vi "Teleop.vi"(10 "Match Info":T1={"Autonomous Elapsed Seconds"=0.0, "TeleOp Elapsed Seconds"=0.0, "Disabled Elapsed Seconds"=0.0, "Visited Autonomous"=FALSE, "Visited TeleOp"=FALSE, "Visited Disabled"=FALSE, "Autonomous Settings"={"Autonomous Style"=enum."Independent", "VI Refnum"=refnum}}, 11 "Call Context":T2) -> ()   [LabVIEW 2016]
doc: "This VI is called for each TeleOp packet received from the DS where the robot is not disabled. It is often used to read from the joysticks and update I/O or to update setpoints for timed control loops. It should complete and return within 20 milliseconds or it may miss DS packets."
uses:
  <vilib>/Rock Robotics/WPI/DriverStation/WPI_DriverStationDerivedRobotMode.ctl
  <vilib>/Rock Robotics/WPI/DriverStation/WPI_DriverStationMatch Info.ctl
  <vilib>/Rock Robotics/WPI/Utilities/WPI_GetSetVariantRefNum.vi
  <vilib>/Rock Robotics/Network Tables/NT Write Boolean Array.vi
  <vilib>/Rock Robotics/Network Tables/NT Write Numeric Array.vi
  <vilib>/Rock Robotics/Network Tables/NT Read Boolean.vi
  <vilib>/Rock Robotics/Network Tables/NT Read Number.vi
  Robot Global Data.vi
  <vilib>/Rock Robotics/WPI/RobotDrive/WPI_RobotDriveArcadeDrive_Standard(NoSaturation).vi
panel:
  out "Sample Slider 0":dbl(slide) scale=0.0..5.0
  out "Sample Boolean 1":bool
  out "Sample Boolean 0":bool
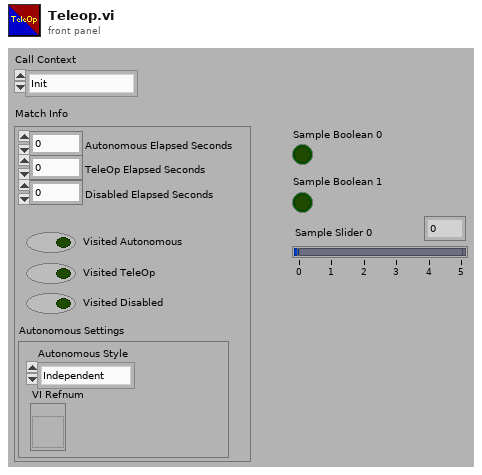
[diagram p1: front panel]
types:
  T1 = typedef "WPI_DriverStationMatch Info.ctl" = cluster{"Autonomous Elapsed Seconds":dbl, "TeleOp Elapsed Seconds":dbl, "Disabled Elapsed Seconds":dbl, "Visited Autonomous":bool, "Visited TeleOp":bool, "Visited Disabled":bool, "Autonomous Settings":cluster{"Autonomous Style":enum16{"Iterative", "Independent"}, "VI Refnum":refnum<vi>}}
  T2 = typedef "WPI_DriverStationDerivedRobotMode.ctl" = enum16{"Init", "Execute", "Stop"}
  T3 = typedef "WPI_JoystickDevRef.ctl" = cluster{"Device":T4}
  T4 = typedef "WPI_JoystickDeviceEnum.ctl" = enum16{"USB 0", "USB 1", "USB 2", "USB 3", "USB 4", "USB 5"}
  T5 = cluster{"Axes[0]":dbl, "Axes[1]":dbl, "Axes[2]":dbl, "Axes[3]":dbl, "Axes[4]":dbl, "Axes[5]":dbl, "Axes[6]":dbl, "Axes[7]":dbl, "Axes[8]":dbl}
  T6 = cluster{"Buttons[0]":bool, "Buttons[1]":bool, "Buttons[2]":bool, "Buttons[3]":bool, "Buttons[4]":bool, "Buttons[5]":bool, "Buttons[6]":bool, "Buttons[7]":bool, "Buttons[8]":bool}
  T7 = typedef "WPI_MotorControlDeviceRef.ctl" = cluster{"DeviceStatus":errorcluster, "Type":T8, "PWM":cluster{"PWM Channel":T9, "DeadBand":T10}, "CAN":cluster{"Device Number":u8, "SetOutput VI Ref":variant, "GetOutput VI Ref":variant, "Enable VI Ref":variant, "Disable VI Ref":variant, "Data":variant}, "Invert":bool}
  T8 = typedef "WPI_MotorControlType.ctl" = enum16{"PWM", "CAN"}
  T9 = typedef "FPGA_DIOPWMChannel.ctl" = enum8{"PWM 0", "PWM 1", "PWM 2", "PWM 3", "PWM 4", "PWM 5", "PWM 6", "PWM 7", "PWM 8", "PWM 9", "PWM MXP 0", "PWM MXP 1", "PWM MXP 2", "PWM MXP 3", "PWM MXP 4", "PWM MXP 5", "PWM MXP 6", "PWM MXP 7", "PWM MXP 8", "PWM MXP 9", "Invalid"}
  T10 = typedef "WPI_PWMDeadband.ctl" = cluster{"Name":string, "maxPositivePwm":i32, "minPositivePwm":i32, "centerPwm":i32, "maxNegativePwm":i32, "minNegativePwm":i32, "angularRange":u16}
  T11 = typedef "WPI_ServoDeviceRef.ctl" = cluster{"DeviceStatus":errorcluster, "PWM Channel":T9, "DeadBand":T10}
  T12 = typedef "WPI_RobotDriveDevRef.ctl" = cluster{"DevStatus":errorcluster, "Motors[]":T7[], "Square Inputs":bool, "Max Output":dbl}
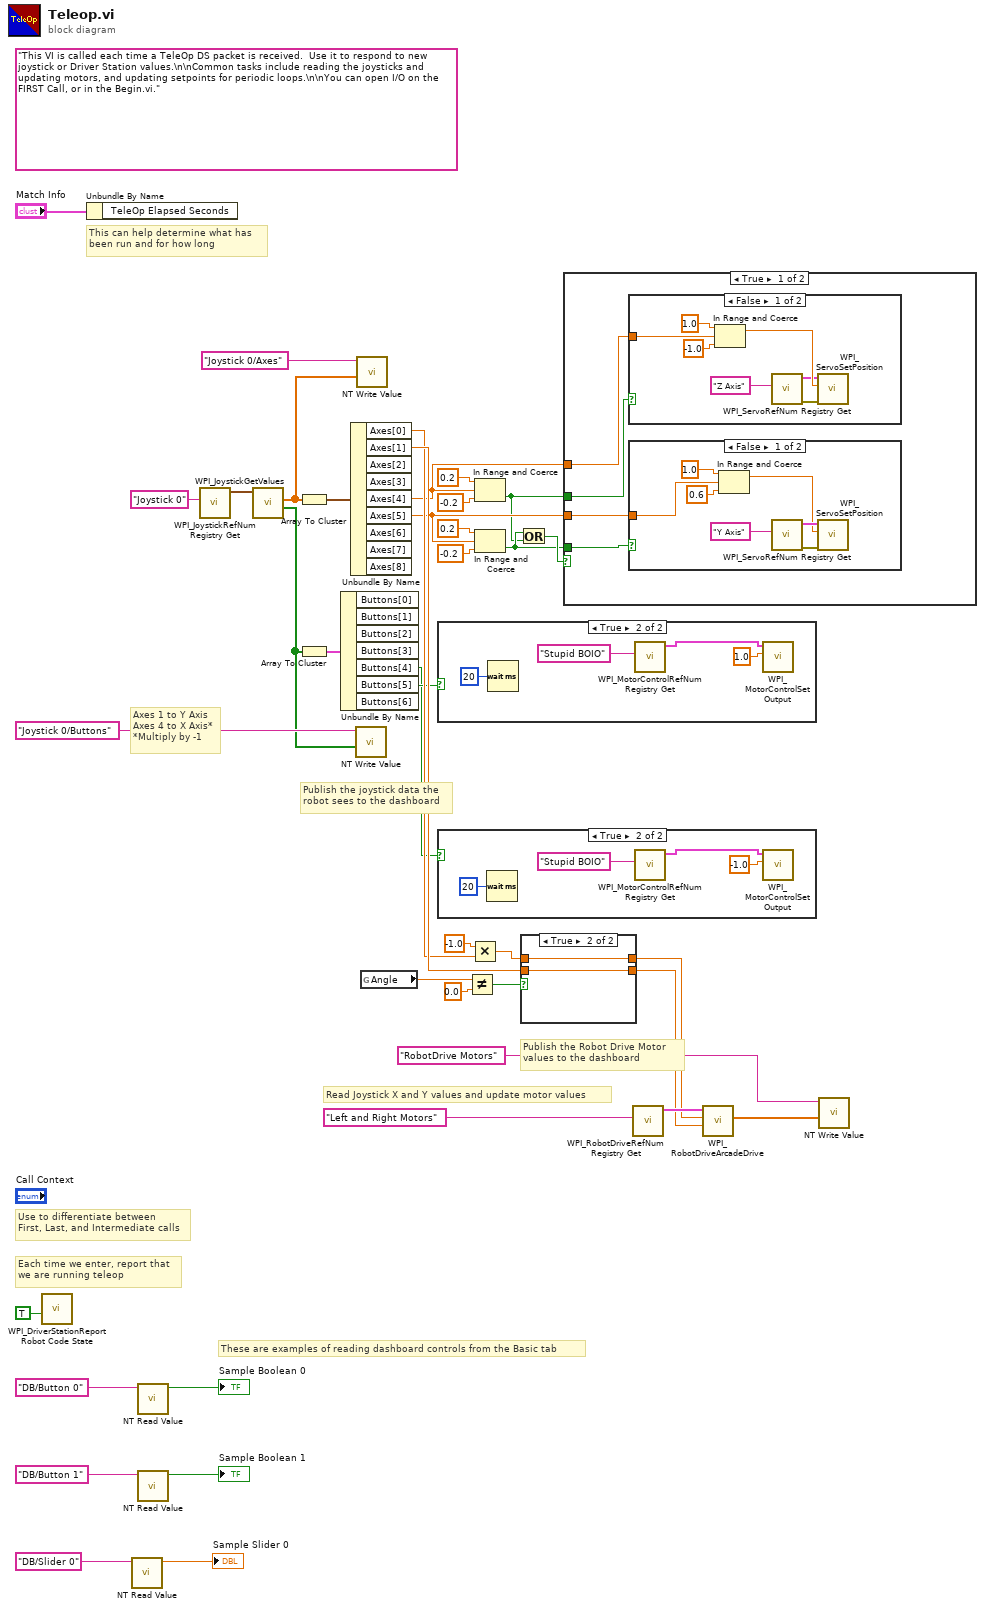
[diagram p0: block diagram]
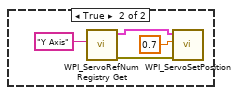
[diagram p4: hidden frame]
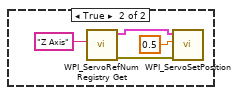
[diagram p5: hidden frame]
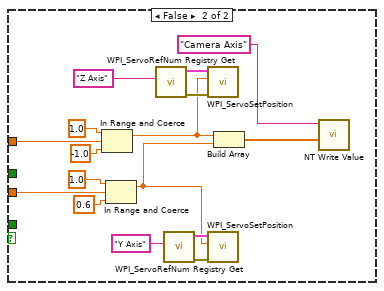
[diagram p6: hidden frame]
diagram:
  (unwired) "This VI is called each time a TeleOp DS packet is received.  Use it to respond to new joystick or Driver Station values.\n\nCommon tasks include reading the joysticks and updating motors, and updating setpoints for periodic loops.\n\nYou can open I/O on the FIRST Call, or in the Begin.vi."
  # "Axes 1 to Y Axis\nAxes 4 to X Axis*\n*Multiply by -1"
  # "These are examples of reading dashboard controls from the Basic tab"
  # "Publish the Robot Drive Motor\nvalues to the dashboard"
  # "Publish the joystick data the\nrobot sees to the dashboard"
  # "Each time we enter, report that\nwe are running teleop"
  # "Use to differentiate between\nFirst, Last, and Intermediate calls"
  # "This can help determine what has\nbeen run and for how long"
  # "Read Joystick X and Y values and update motor values"
  n1 = call <vilib>:"WPI_DriverStationReport Robot Code State.vi"("TeleOp"=TRUE ("Autonomous")) -> ()  [unwired: 10 in, 1 out]
  n2 = Unbundle By Name("Match Info") -> ()  [unwired: 1 out]
  n3 = call-poly <vilib>:"NT Read Value.vi"("Name"="DB/Slider 0" ("refnum name")) -> ("Numeric"=→"Sample Slider 0":dbl)  [unwired: 9 in, 1 out]
  n4 = call-poly <vilib>:"NT Read Value.vi"("Name"="DB/Button 0" ("refnum name")) -> ("Boolean"=→"Sample Boolean 0":bool)  [unwired: 9 in, 1 out]
  n5 = call-poly <vilib>:"NT Read Value.vi"("Name"="DB/Button 1" ("refnum name")) -> ("Boolean"=→"Sample Boolean 1":bool)  [unwired: 9 in, 1 out]
  n6 = call <vilib>:"WPI_JoystickRefNum Registry Get.vi"("refnum name"="Joystick 0") -> ("JoystickDevRef"=w37:T3)  [unwired: 1 in, 9 out]
  n7 = call <vilib>:"WPI_JoystickGetValues.vi"("JoystickDevRef"=w37) -> ("Buttons"=w4:bool[], "Axes"=w23:dbl[])  [unwired: 6 in, 3 out]
  n8 = Array To Cluster(array=w23) -> (cluster=w26:T5)
  n9 = Array To Cluster(array=w4) -> (cluster=w3:T6)
  n10 = Unbundle By Name(w3) -> ("Buttons[4]"=w1:bool, "Buttons[5]"=w2:bool)  [unwired: 5 out]
  n11 = Unbundle By Name(w26) -> ("Axes[0]"=w16:dbl, "Axes[1]"=w19:dbl, "Axes[4]"=w10:dbl, "Axes[5]"=w13:dbl)  [unwired: 5 out]
  n12 = call-poly <vilib>:"NT Write Value.vi"("Boolean Array"=w4, "Name"="Joystick 0/Buttons") -> ()  [unwired: 9 in, 1 out]
  n13 = call-poly <vilib>:"NT Write Value.vi"("Numeric Array"=w23, "Name"="Joystick 0/Axes") -> ()  [unwired: 9 in, 1 out]
  n14 = global read "Robot Global Data.vi" "Angle"() -> (w22:dbl)
  n15 = case shown="True" w2 {
    frame False {
    }
    frame True {
      n16 = Wait (ms)(milliseconds to wait=u32 20) -> ()  [unwired: 1 out]
      n17 = call <vilib>:"WPI_MotorControlRefNum Registry Get.vi"("refnum name"="Stupid BOIO") -> ("MotorControlDevRef"=w44:T7)  [unwired: 9 in, 1 out]
      n18 = call <vilib>:"WPI_MotorControlSetOutput.vi"("Output"=1.0, "MotorControlDevRef"=w44) -> ()  [unwired: 7 in, 3 out]
    }
  }
  n19 = case shown="True" w1 {
    frame False {
    }
    frame True {
      n20 = Wait (ms)(milliseconds to wait=u32 20) -> ()  [unwired: 1 out]
      n21 = call <vilib>:"WPI_MotorControlRefNum Registry Get.vi"("refnum name"="Stupid BOIO") -> ("MotorControlDevRef"=w48:T7)  [unwired: 9 in, 1 out]
      n22 = call <vilib>:"WPI_MotorControlSetOutput.vi"("Output"=-1.0, "MotorControlDevRef"=w48) -> ()  [unwired: 7 in, 3 out]
    }
  }
  n23 = Not Equal?(x=w22, y=0.0) -> (x != y?=w20:bool)
  n24 = Multiply(x=-1.0 ("y"), y=w16) -> (x*y=w15:dbl)
  n25 = In Range and Coerce(upper limit=0.2, x=w10, lower limit=-0.2) -> (In Range?=w5:bool)  [unwired: 1 out]
  n26 = In Range and Coerce(upper limit=0.2, x=w13, lower limit=-0.2) -> (In Range?=w6:bool)  [unwired: 1 out]
  n27 = Or(x=w6, y=w5) -> (x .or. y?=w7:bool)
  n28 = case shown="True" w20 {
    tunnel: w19 -> [w50 w52]
    tunnel: [w50 w52] -> w18
    tunnel: [w49 w51] -> w17
    tunnel: w15 -> [w49 w51]
    frame False {
    }
    frame True {
    }
  }
  n29 = case shown="True" w7 {
    tunnel: w10 -> [w54 w86]
    tunnel: w13 -> [w53 w83]
    tunnel: w6 -> [w56 _]
    tunnel: w5 -> [w55 _]
    frame True {
      n30 = case shown="False" w55 {
        tunnel: w54 -> [w69 _]
        frame False {
          n31 = In Range and Coerce(upper limit=1.0, x=w69, lower limit=-1.0) -> (coerced(x)=w72:dbl)  [unwired: 1 out]
          n32 = call <vilib>:"WPI_ServoRefNum Registry Get.vi"("refnum name"="Z Axis") -> ("error out"=w68:errorcluster, "ServoDeviceRef"=w70:T11)  [unwired: 9 in]
          n33 = call <vilib>:"WPI_ServoSetPosition.vi"("error in (no error)"=w68, "Position"=w72, "ServoDeviceRef"=w70) -> ()  [unwired: 7 in, 2 out]
        }
        frame True {
          n34 = call <vilib>:"WPI_ServoRefNum Registry Get.vi"("refnum name"="Z Axis") -> ("error out"=w77:errorcluster, "ServoDeviceRef"=w76:T11)  [unwired: 9 in]
          n35 = call <vilib>:"WPI_ServoSetPosition.vi"("error in (no error)"=w77, "Position"=0.5, "ServoDeviceRef"=w76) -> ()  [unwired: 7 in, 2 out]
        }
      }
      n36 = case shown="False" w56 {
        tunnel: w53 -> [w57 _]
        frame False {
          n37 = In Range and Coerce(upper limit=1.0, x=w57, lower limit=0.6) -> (coerced(x)=w60:dbl)  [unwired: 1 out]
          n38 = call <vilib>:"WPI_ServoRefNum Registry Get.vi"("refnum name"="Y Axis") -> ("error out"=w63:errorcluster, "ServoDeviceRef"=w62:T11)  [unwired: 9 in]
          n39 = call <vilib>:"WPI_ServoSetPosition.vi"("error in (no error)"=w63, "Position"=w60, "ServoDeviceRef"=w62) -> ()  [unwired: 7 in, 2 out]
        }
        frame True {
          n40 = call <vilib>:"WPI_ServoRefNum Registry Get.vi"("refnum name"="Y Axis") -> ("error out"=w66:errorcluster, "ServoDeviceRef"=w65:T11)  [unwired: 9 in]
          n41 = call <vilib>:"WPI_ServoSetPosition.vi"("error in (no error)"=w66, "Position"=0.7, "ServoDeviceRef"=w65) -> ()  [unwired: 7 in, 2 out]
        }
      }
    }
    frame False {
      n42 = In Range and Coerce(upper limit=1.0, x=w86, lower limit=-1.0) -> (coerced(x)=w85:dbl)  [unwired: 1 out]
      n43 = In Range and Coerce(upper limit=1.0, x=w83, lower limit=0.6) -> (coerced(x)=w84:dbl)  [unwired: 1 out]
      n44 = call <vilib>:"WPI_ServoRefNum Registry Get.vi"("refnum name"="Z Axis") -> ("error out"=w92:errorcluster, "ServoDeviceRef"=w91:T11)  [unwired: 9 in]
      n45 = call <vilib>:"WPI_ServoRefNum Registry Get.vi"("refnum name"="Y Axis") -> ("error out"=w88:errorcluster, "ServoDeviceRef"=w89:T11)  [unwired: 9 in]
      n46 = call <vilib>:"WPI_ServoSetPosition.vi"("error in (no error)"=w92, "Position"=w85, "ServoDeviceRef"=w91) -> ()  [unwired: 7 in, 2 out]
      n47 = call <vilib>:"WPI_ServoSetPosition.vi"("error in (no error)"=w88, "Position"=w84, "ServoDeviceRef"=w89) -> ()  [unwired: 7 in, 2 out]
      n48 = Build Array(w85, w84) -> (w94:dbl[])
      n49 = call-poly <vilib>:"NT Write Value.vi"("Numeric Array"=w94, "Name"="Camera Axis") -> ()  [unwired: 9 in, 1 out]
    }
  }
  n50 = call <vilib>:"WPI_RobotDriveRefNum Registry Get.vi"("refnum name"="Left and Right Motors") -> ("RobotDriveDevRef"=w24:T12)  [unwired: 1 in, 9 out]
  n51 = call-poly <vilib>:"WPI_RobotDriveArcadeDrive.vi"("Y axis value"=w18, "X axis value"=w17, "RobotDriveDevRef"=w24) -> ("Motor Values"=w25:dbl[])  [unwired: 6 in, 2 out]
  n52 = call-poly <vilib>:"NT Write Value.vi"("Numeric Array"=w25, "Name"="RobotDrive Motors") -> ()  [unwired: 9 in, 1 out]
